vi "read msg.vi"(8 "error in (no error)":errorcluster) -> (0 "error out":errorcluster, 3 "信息簇":T1 {"采样模式选择" items=["定时留样", "时间等比例", "同步留样", "外控留样", "超标留样"]; "启停" items=["停止", "启动"]; "采样器进程" items=["待机"=1, "采样瓶排空"=2, "采样瓶润洗"=5, "进样"=6, "取样"=8, "取样管排空"=9]; "门禁标志" items=["关闭", "打开"]; "远程留样" items=["停止", "留样"]})   [LabVIEW 2016, in "DR803M4.lvlib"]
uses:
  DR803M4.lvlib
  <vilib>/Plasmionique/MB Master/MB_Master_Serial/MB_Master_Serial.lvclass
  C:/Program Files (x86)/National Instruments/LabVIEW 2016/vi.lib/Plasmionique/MB Master/MB_Master/MB_Master.lvclass
  Global variable/input variable.vi
  <vilib>/Plasmionique/MB Master/MB Master.lvlib
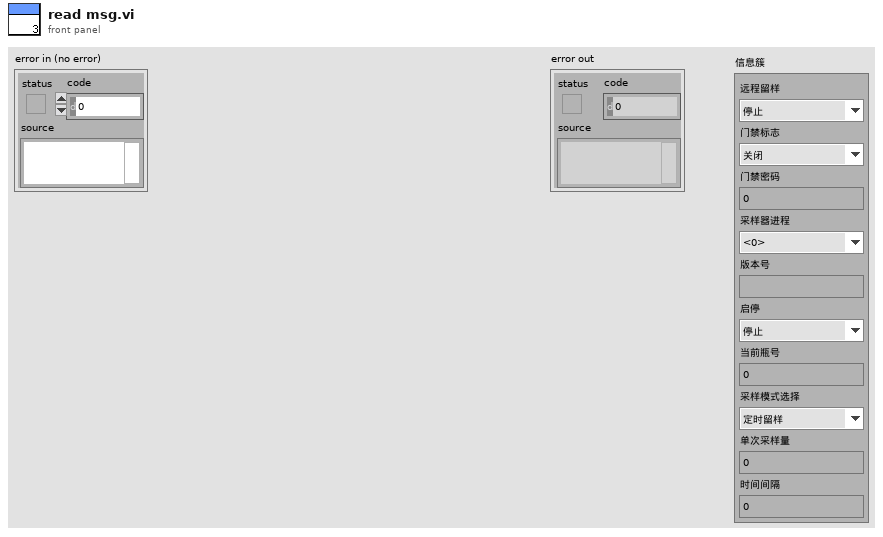
[diagram p1: front panel]
types:
  T1 = cluster{"远程留样":u16, "门禁标志":u16, "门禁密码":u32, "采样器进程":u16, "版本号":string, "启停":u16, "当前瓶号":u16, "采样模式选择":u16, "单次采样量":u16, "时间间隔":u16}
  T2 = cluster{u16, u16, u32, u16, string, u16, u16, u16, u16, u16}
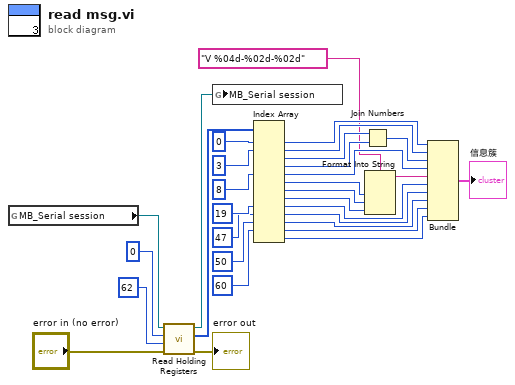
[diagram p0: block diagram]
diagram:
  n1 = global read "input variable.vi" "MB_Serial session"() -> (w31:refnum<class "MB_Master_Serial.lvclass">)
  n2 = call <vilib>:"Read Holding Registers.vi"("error in (no error)"="error in (no error)", "quantity"=u16 62, "starting address"=u16 0, "MB session in"=w31) -> ("error out"=→"error out":errorcluster, "Registers"=w25:u16[], "MB session out"=w26:refnum<class "MB_Master_Serial.lvclass">)  [unwired: 5 in]
  n3 = global write "input variable.vi" "MB_Serial session"(w26) -> ()
  n4 = Index Array(array=w25, index #1=0 ("索引"), index #2=3 ("索引"), index #5=8 ("索引"), index #9=19 ("索引"), index #10=47 ("索引"), index #11=50 ("索引"), index #12=60 ("索引")) -> (element #1=w15:u16, element #2=w14:u16, element #3=w22:u16, element #4=w21:u16, element #5=w12:u16, element #6=w5:u16, element #7=w4:u16, element #8=w3:u16, element #9=w11:u16, element #10=w10:u16, element #11=w9:u16, element #12=w8:u16, element #13=w7:u16)  [unwired: 6 in]
  n5 = Join Numbers(hi=w22, lo=w21) -> ((hi.lo)=w13:u32)
  n6 = Format Into String(format string="V %04d-%02d-%02d" ("格式字符串"), w5, w4, w3) -> (resulting string=w2:string)  [unwired: 2 in, 1 out]
  n7 = Bundle(w15, w14, w13, w12, w2, w11, w10, w9, w8, w7) -> (→"信息簇":T2)  [unwired: 1 in]
